vi "SetpointArrays.vi"(10 "Setpoint2":dbl, 11 "Setpoint1":dbl) -> (3 "Motor Setpoints":dbl[](array[numeric]))   [LabVIEW 2014]
panel:
  # "This one only works for doubles"
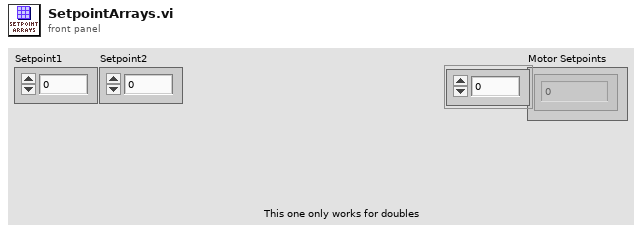
[diagram p1: front panel]
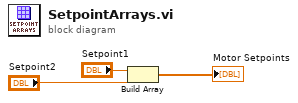
[diagram p0: block diagram]
diagram:
  n1 = Build Array("Setpoint1", "Setpoint2") -> (→"Motor Setpoints":dbl[])
